vi "TF_Tacho2Velocity.vi"(2 "Motor Velocity Tacho Value [V]":dbl) -> (5 "Motor Velocity Tacho [deg/s]":dbl)   [LabVIEW 2019]
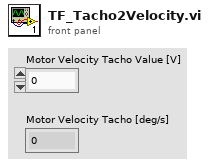
[diagram p1: front panel]
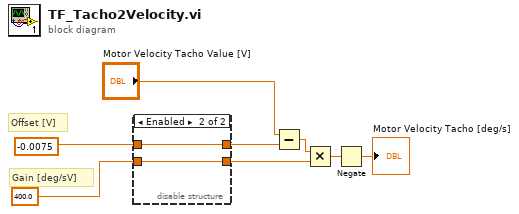
[diagram p0: block diagram]
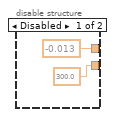
[diagram p2: hidden frame]
diagram:
  # "Gain [deg/sV]"
  # "Offset [V]"
  n1 = disable-structure shown="Enabled" {
    disable-tunnel: [300.0 ("gain") w11] -> w8
    disable-tunnel: [-0.013 ("offset") w12] -> w6
    disable-tunnel: -0.0075 -> [_ w12]
    disable-tunnel: 400.0 -> [_ w11]
    frame Disabled {
    }
    frame Enabled {
    }
  }
  n2 = Subtract(x="Motor Velocity Tacho Value [V]", y=w6) -> (x-y=w4:dbl)
  n3 = Multiply(x=w4, y=w8) -> (x*y=w7:dbl)
  n4 = Negate(x=w7) -> (-x=→"Motor Velocity Tacho [deg/s]":dbl)
